vi "ziModExecute.vi"(7 "Error In":errorcluster, 9 "Modal (F)":bool, 10 "ziModHandle In":T1 {"ModHandle" format="0x%08x"; "Conn" format="0x%08x"}) -> (0 "Error Out":errorcluster, 3 "ziModHandle Out":T1 {"ModHandle" format="0x%08x"; "Conn" format="0x%08x"})   [LabVIEW 2009, in "Zurich Instruments LabOne.lvlib"]
doc: "Start the module. If the <b>Modal</b> is set to false, the vi waits for the module to finish and polls the data from the device. Use ziModGetNextNode.vi in order to access the availible data. If the <b>Modal</b> is set to true, the module is started. In order to poll the data from the device use ziModRead.vi."
uses:
  <instrlib>/Zurich Instruments LabOne/Zurich Instruments LabOne.lvlib
  <instrlib>/Zurich Instruments LabOne/Public/Modules/ziTypeModHandle.ctl
panel:
  out "Finished?":bool
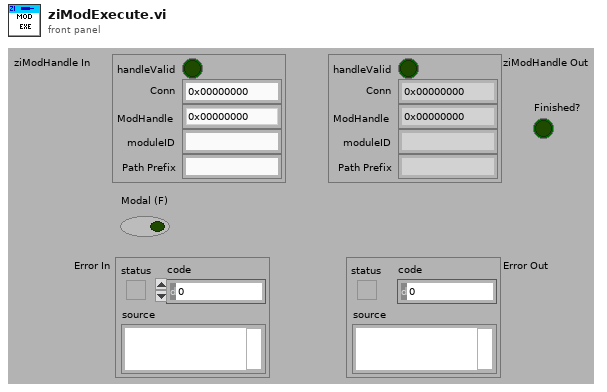
[diagram p1: front panel]
types:
  T1 = typedef "Zurich Instruments LabOne.lvlib/ziTypeModHandle.ctl" = cluster{"handleValid":bool, "Conn":u64, "ModHandle":u64, "moduleID":string, "Path Prefix":string}
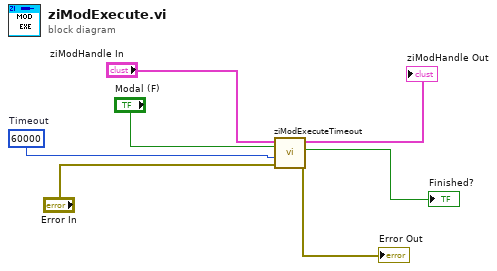
[diagram p0: block diagram]
diagram:
  w5 = u32 60000  # Timeout
  n1 = call <instrlib>:"ziModExecuteTimeout.vi"("Error In"="Error In", "Timeout 5000ms"=w5, "Modal (F)"="Modal (F)", "ziModHandle In"="ziModHandle In") -> ("Error Out"=→"Error Out":errorcluster, "Finished?"=→"Finished?":bool, "ziModHandle Out"=→"ziModHandle Out":T1)  [unwired: 4 in]
